vi "LVClass_CorrectionDataManager GetGreatestCommonPupil.vi"(0 "CorrectionDataManager in":refnum<class "CorrectionDataManager.lvclass">, 5 "Pupil in":refnum<class "Pupil.lvclass">, 11 "error in (no error)":errorcluster) -> (4 "CorrectionDataManager out":refnum<class "CorrectionDataManager.lvclass">, 6 "Pupil out":refnum<class "Pupil.lvclass">, 15 "error out":errorcluster)   [LabVIEW 2020, in "CorrectionDataManager.lvclass"]
doc: "Computes the greatest common pupil.\n\n--------------------------------------------------------------------------------\n\n<B>corrdata_managerIn </B> : CorrDataManager object.\n<B>corrdata_managerOut </B> : CorrDataManager object.\n<B>pupil </B> : Greatest common pupil as a 2D Array\n<B>ErrorIn </B> : Error\n<B>ErrorOut </B> : Error\n\n--------------------------------------------------------------------------------"
uses:
  CorrectionDataManager.lvclass
  Pupil.lvclass
  CorrectionDataManager.lvclass/CorrectionDataManager.ctl
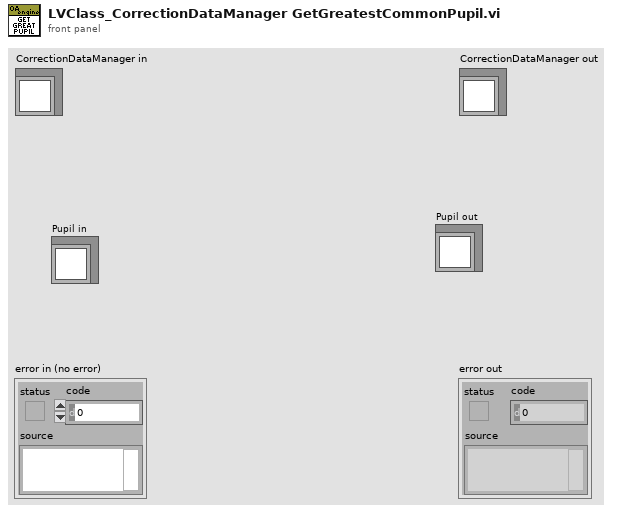
[diagram p1: front panel]
types:
  T1 = typedef "General dimensions definition.ctl" = cluster{"Size":T2, "Step":T3}
  T2 = typedef "Point2D.ctl" = cluster{"X":u32, "Y":u32}
  T3 = typedef "Point2Df.ctl" = cluster{"X":sgl, "Y":sgl}
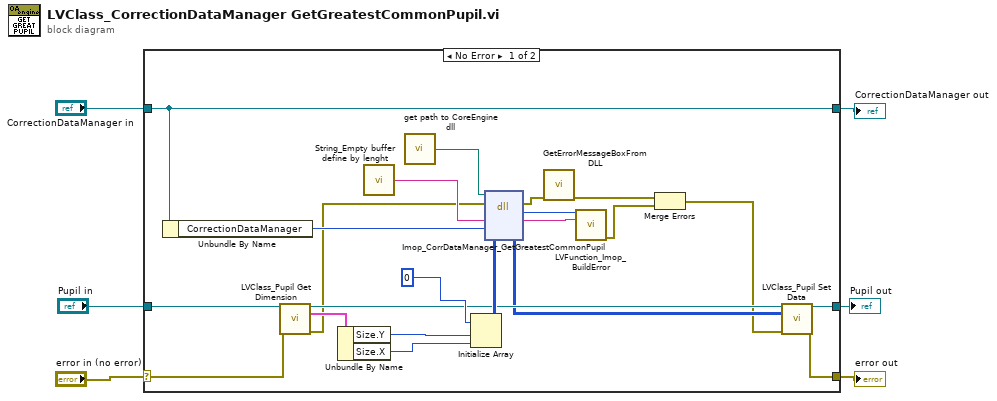
[diagram p0: block diagram]
diagram:
  n1 = case shown="No Error" "error in (no error)" {
    selector: "error in (no error)" -> [w10 w31]
    tunnel: [w7 w31] -> w4
    tunnel: [w21 w30] -> w5
    tunnel: "CorrectionDataManager in" -> [w21 w30]
    tunnel: "Pupil in" -> [w19 w29]
    tunnel: [w9 w29] -> w1
    frame No Error {
      n2 = Unbundle By Name(w21) -> ("CorrectionDataManager"=w20:i32)
      n3 = call "LVClass_Pupil Get Dimension.vi"("Pupil in"=w19, "error in (no error)"=w10) -> ("Pupil out"=w13:refnum<class "Pupil.lvclass">, "Dimension"=w18:T1, "error out"=w11:errorcluster)  [unwired: 11 in]
      n4 = Unbundle By Name(w18) -> ("Size.Y"=w16:u32, "Size.X"=w15:u32)
      n5 = call "String_Empty buffer define by lenght.vi"() -> ("Empty buffer"=w26:string)  [unwired: 1 in]
      n6 = call "get path to CoreEngine dll.vi"() -> ("path to c_interface_vc100.dll"=w22:path)  [unwired: 12 in, 3 out]
      n7 = Initialize Array(u8 0, w16, w15) -> (w14:u8[][])
      n8 = dll-call lib="D:/soft/HASO_v3/SVN_trunk/ImOpCoreEngine4_LV2011/DLLs/c_interface_vc100.dll" fn="Imop_CorrDataManager_GetGreatestCommonPupil"(path in=w22, error in=w11, "message"=w26, "corrdata_manager"=w20, "pupil"=w14) -> (error out=w25:errorcluster, "return type"=w28:i32, "message"=w27:string, "pupil"=w12:u8[][])  [unwired: 2 in, 1 out]
      n9 = call "GetErrorMessageBoxFromDLL.vi"("error IN"=w25) -> ("error OUT"=w24:errorcluster)  [unwired: 10 in]
      n10 = call "LVFunction_Imop_BuildError.vi"("code"=w28, "String to Prepend to source (\"\")"=w27) -> ("error out"=w23:errorcluster)  [unwired: 13 in]
      n11 = Merge Errors(w24, w23) -> (w8:errorcluster)
      n12 = call "LVClass_Pupil Set Data.vi"("Pupil in"=w13, "Data"=w12, "error in (no error)"=w8) -> ("Pupil out"=w9:refnum<class "Pupil.lvclass">, "error out"=w7:errorcluster)  [unwired: 11 in]
    }
    frame Error {
    }
  }
  "error out" <- w4
  "CorrectionDataManager out" <- w5
  "Pupil out" <- w1
